vi "Wait Until Settled.vi"(0 "device session in":refnum<class "Device Session.lvclass">, 11 "error in":errorcluster) -> (4 "device session out":refnum<class "Device Session.lvclass">, 15 "error out":errorcluster)   [LabVIEW 2021, in "Device Session.lvclass"]
doc: "Waits until the device analog input circuitry settles. Call this VI after configuring the channel to wait for the input circuitry to settle.\n\n<B>Input Parameters</B>\n\n<B>device session in</B> is a reference to the Device Session object, which contains a session to each instrument design library used in this sample project. This parameter is obtained from the 'Open Session' VI.\n\n<B>error in</B> describes error conditions that occur before this node runs. This input provides standard 'error in' functionality.\n\n<B>Output Parameters</B>\n\n<B>device session out</B> passes a reference to the session to the next VI.\n\n<B>error out</B> contains error information. This output provides standard 'error out' functionality."
uses:
  Device Session.lvclass
  Device Session.lvclass/Device Session.ctl
  <instrlib>/HSAI-RIO/Config/Group A/v1/Host/Main/niHSAI Group A Config v1 Host.lvclass
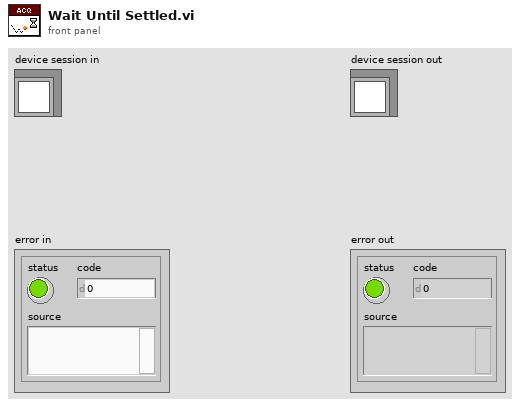
[diagram p1: front panel]
types:
  T1 = typedef "Device Session.lvclass/Device Session Object.ctl" = cluster{"fpga reference":T2, "reg bus":refnum<class "niInstr FIFO Register Bus v1 Host.lvclass">, "subsystem map":refnum<class "niInstr Subsystem Map v1 Host.lvclass">, "cal data":refnum<class "niHSAI Cal Data v1 Host.lvclass">, "config":refnum<class "niHSAI Group A Config v1 Host.lvclass">, "acquisition":refnum<class "niInstr Multirecord Acquisition v1 Host.lvclass">, "number of selected acq channels":u8, "selected acq channels":bool[], "number of channels":u32, "configured channels":bool[], "acq configuration":cluster{"number of samples":u64, "number of records":u64, "pretrigger samples":u64}, "actual channel configuration":T3[], "sample clock rate (Hz)":dbl, "scaling coefficients":T7[]}
  T2 = typedef "Device Session.lvclass/FPGA Refnum.ctl" = refnum<k20>
  T3 = typedef "niHSAI Types v1 Host.lvlib/Channel Configuration.ctl" = cluster{"channel":u32, "coupling":T4, "impedance":T5, "bandwidth":T6, "vertical range":dbl, "vertical offset":dbl}
  T4 = typedef "niHSAI Types v1 Host.lvlib/Coupling.ctl" = enum8{"Default", "DC", "AC"}
  T5 = typedef "niHSAI Types v1 Host.lvlib/Impedance.ctl" = enum8{"Default", "1 mega ohm", "50 ohm"}
  T6 = typedef "niHSAI Types v1 Host.lvlib/Bandwidth.ctl" = enum8{"Default", "Full Bandwidth", "Anti-alias Filter", "150 MHz"}
  T7 = typedef "niInstr Multirecord Acquisition v1 Host.lvclass/Scaling Coefficient.ctl" = cluster{"gain":dbl, "offset":dbl}
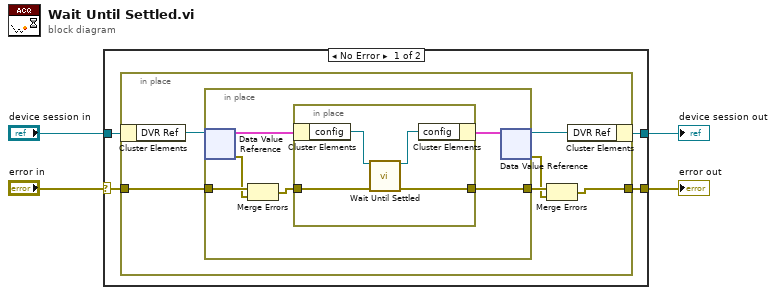
[diagram p0: block diagram]
diagram:
  n1 = case shown="No Error" "error in" {
    selector: "error in" -> [w8 w26]
    tunnel: "device session in" -> [w6 w25]
    tunnel: [w5 w25] -> w2
    tunnel: [w7 w26] -> w1
    frame No Error {
      n2 = in-place {
        in-place-border: w8 -> [w14]
        in-place-border: [w9] -> w7
        n3 = in-place-cluster #1(w6) -> ("DVR Ref"=w11:refnum<data-value>)
        n4 = in-place {
          in-place-border: w14 -> [w19]
          in-place-border: [w20] -> w13
          n5 = in-place-dvr #2(w11) -> (w16:T1, w18:errorcluster)
          n6 = Merge Errors(w19, w18) -> (w17:errorcluster)
          n7 = in-place {
            in-place-border: [w24] -> w20
            in-place-border: w17 -> [w23]
            n8 = in-place-cluster #3(w16) -> ("config"=w22:refnum<class "niHSAI Group A Config v1 Host.lvclass">)
            n9 = call-dynamic "Wait Until Settled.vi"("session in"=w22, "error in"=w23) -> ("session out"=w21:refnum<class "niHSAI Group A Config v1 Host.lvclass">, "error out"=w24:errorcluster)  [unwired: 12 in]
            n10 = in-place-cluster #3("config"=w21) -> (w15:T1)
          }
          n11 = in-place-dvr #2(w15) -> (w10:refnum<data-value>, w12:errorcluster)
        }
        n12 = Merge Errors(w13, w12) -> (w9:errorcluster)
        n13 = in-place-cluster #1("DVR Ref"=w10) -> (w5:refnum<class "Device Session.lvclass">)
      }
    }
    frame Error {
    }
  }
  "error out" <- w1
  "device session out" <- w2
